vi "Input Entry.vi"(8 "error in (no error)":errorcluster, 9 "Project In":refnum<class "Project.lvclass">, 11 "Input Control":T2) -> (0 "error out":errorcluster)   [LabVIEW 2015, in "CallVIStep.lvclass"]
uses:
  CallVIStep.lvclass
  VI Input Control Typedef.ctl
  VI Input Type Typedef.ctl
  Project.lvclass
  SerializableObject/CONFIGURE_UI_STATE.ctl
  Editor/Editor.lvclass
panel:
  in  "Unsupport Type":string caption="_STRING"
  in  "Variable Name":string(combo)
  in  "Input Type":T1
  in  "_DAQmx":refnum<k21>
  in  "_COMBO_BOX":string(combo)
  in  "_ENUM":enum16{""}(ring)
  in  "_VISA":refnum<visa-resource-name>
  in  "_COLOR_BOX":u32(colorbox)
  in  "_RING":u16(ring)=5 items=["Text"=5, "ColorBox"=7, "Path"=11, "Numeric"=17, "Digital"=18, "String"=27, "IOName"=28, "ComboBox"=29, "Enum"=35, "DAQName"=49, "VISAName"=50]
  in  "_BOOLEAN":bool
  in  "_PATH":path
  in  "_NUMERIC":dbl
  in  "_STRING":string
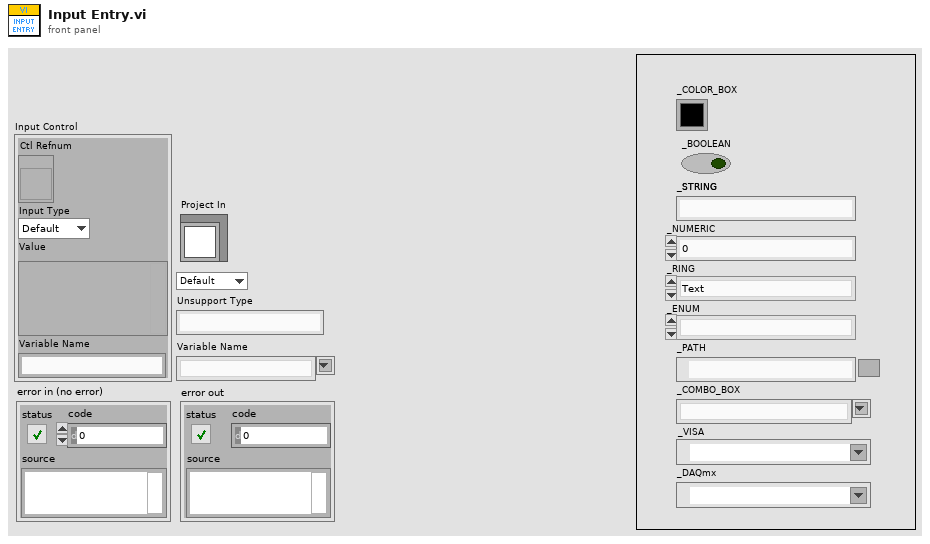
[diagram p1: front panel]
types:
  T1 = typedef "CallVIStep.lvclass/VI Input Type Typedef.ctl" = enum16{"Default", "Value", "Variable"}
  T2 = typedef "CallVIStep.lvclass/VI Input Control Typedef.ctl" = cluster{"Ctl Refnum":refnum<vi>, "Input Type":T1, "Value":variant, "Variable Name":string}
  T3 = cluster{"VI Refnum":refnum<vi>, "Input Type Refnum":refnum<vi>, "Variable Name Refnum":refnum<vi>, "Unsupport Type Refnum":refnum<vi>}
  T4 = typedef "Editor.lvclass/CONFIGURE_UI_STATE.ctl" = enum16{"UI_LOOP", "INIT", "END", "CHANGE_PANEL"}
  T5 = typedef "LVRectTypeDef.ctl" = cluster{"Left":i16, "Top":i16, "Right":i16, "Bottom":i16}
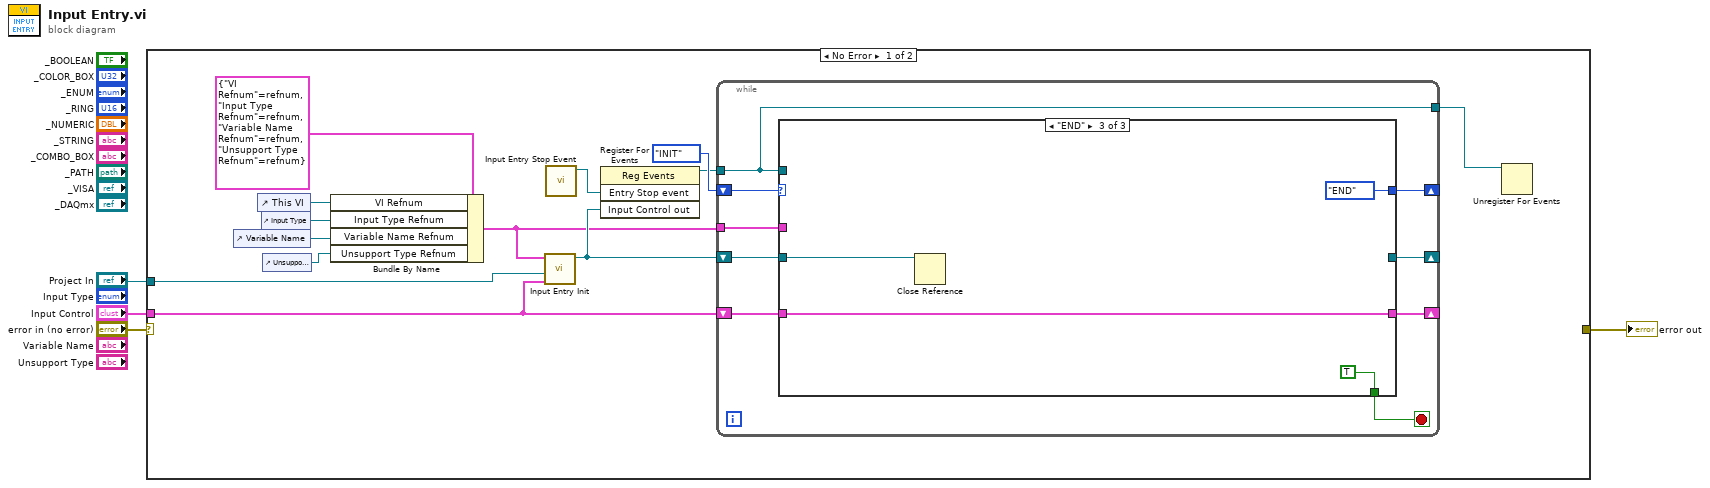
[diagram p0: block diagram]
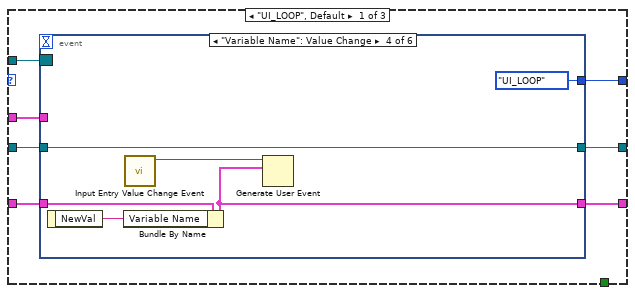
[diagram p2: hidden frame]
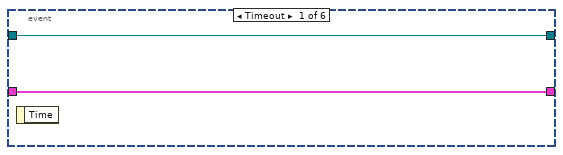
[diagram p3: hidden frame]
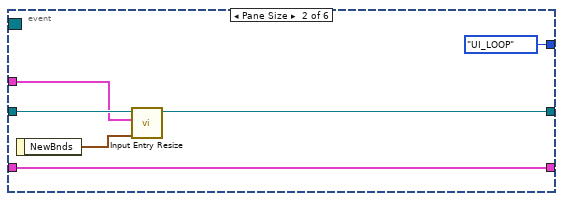
[diagram p4: hidden frame]
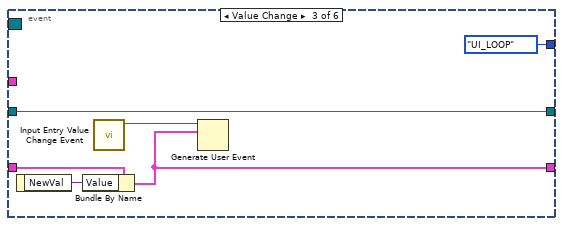
[diagram p5: hidden frame]
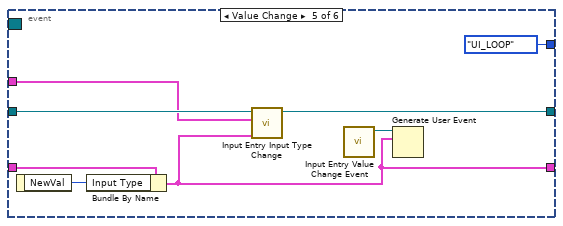
[diagram p6: hidden frame]
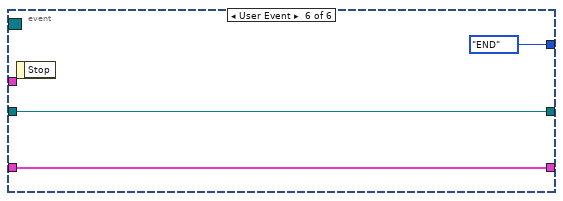
[diagram p7: hidden frame]
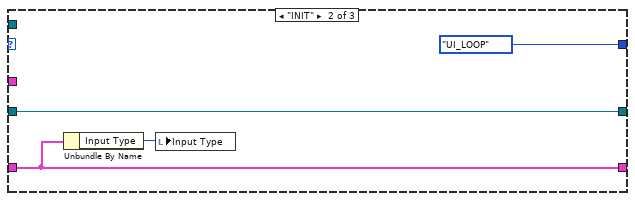
[diagram p8: hidden frame]
diagram:
  n1 = case shown="No Error" "error in (no error)" {
    selector: "error in (no error)" -> [_ w73]
    tunnel: [_ w73] -> w3
    tunnel: "Input Control" -> [w11 _]
    tunnel: "Project In" -> [w12 _]
    frame No Error {
      n2 = control-ref of="Variable Name"() -> (w7:refnum<vi>)
      n3 = control-ref of="This VI"() -> (w9:refnum<vi>)
      n4 = control-ref of="Input Type"() -> (w8:refnum<vi>)
      n5 = control-ref of="Unsupport Type"() -> (w6:refnum<vi>)
      n6 = Bundle By Name(cluster=T3 {"VI Refnum"=refnum, "Input Type Refnum"=refnum, "Variable Name Refnum"=refnum, "Unsupport Type Refnum"=refnum} ("Refnums"), "VI Refnum"=w9, "Input Type Refnum"=w8, "Variable Name Refnum"=w7, "Unsupport Type Refnum"=w6) -> (w5:T3)
      n7 = call "Input Entry Init.vi"("Input Control"=w11, "Project In"=w12, "Refnums"=w5) -> ("Input Control out"=w13:refnum<vi>)  [unwired: 8 in]
      n8 = call "Input Entry Stop Event.vi"() -> ("Entry Stop event"=w16:refnum<user-event>)  [unwired: 11 in]
      n9 = register-events(w16, w13) -> (reference out=w15:refnum<event-registration>)  [unwired: 2 in, 1 out]
      n10 = while {
        shift-right: [w25] -> _
        shift-left: CONFIGURE_UI_STATE."INIT" -> [w26]
        tunnel: w15 -> [w22]
        tunnel: [w22] -> w14
        shift-right: [w20] -> _
        shift-left: w13 -> [w21]
        shift-right: [w19] -> _
        shift-left: w11 -> [w23]
        tunnel: w5 -> [w18]
        stop <- w24 stop-if-true
        n11 = case shown="\"END\"" w26 {
          tunnel: [w33 CONFIGURE_UI_STATE."UI_LOOP" CONFIGURE_UI_STATE."END"] -> w25
          tunnel: [_ _ TRUE] -> w24
          tunnel: w23 -> [w29 w65 w69]
          tunnel: w22 -> [w32 _ _]
          tunnel: w21 -> [w31 w67 w70]
          tunnel: [w30 w67 _] -> w20
          tunnel: [w28 w65 w69] -> w19
          tunnel: w18 -> [w27 _ _]
          frame "UI_LOOP", Default {
            n12 = event shown="[3] \"Variable Name\": Value Change" {
              selector: w32 -> [_ _ _ _ _ _]
              dyn-events: _ -> [_ _ _ _ _ _]
              timeout: _ -> [_ _ _ _ _ _]
              tunnel: [_ CONFIGURE_UI_STATE."UI_LOOP" CONFIGURE_UI_STATE."UI_LOOP" CONFIGURE_UI_STATE."UI_LOOP" CONFIGURE_UI_STATE."UI_LOOP" CONFIGURE_UI_STATE."END"] -> w33
              tunnel: w31 -> [w35 w41 w47 w53 w59 w63]
              tunnel: [w35 w40 w47 w53 w58 w63] -> w30
              tunnel: w29 -> [w34 w37 w46 w52 w56 w62]
              tunnel: [w34 w37 w42 w48 w55 w62] -> w28
              tunnel: w27 -> [_ w36 _ _ w54 _]
              event Timeout {
                n13 = event-data() -> ()  [unwired: 1 in, 1 out]
              }
              event Pane Size {
                n14 = event-data() -> ("NewBnds"=w38:T5)  [unwired: 1 in]
                n15 = call "Input Entry Resize.vi"("NewBnds"=w38, "Refnums"=w36, "Control Refnum in"=w41) -> ("Control Refnum out"=w40:refnum<vi>)  [unwired: 8 in]
              }
              event Value Change {
                n16 = event-data() -> ("NewVal"=w45:variant)  [unwired: 1 in]
                n17 = Bundle By Name(cluster=w46, "Value"=w45) -> (w42:T2)
                n18 = call "Input Entry Value Change Event.vi"() -> ("Entry Value Change Event"=w44:refnum<user-event>)  [unwired: 11 in]
                n19 = Generate User Event(user event=w44, event data cluster=w42) -> ()  [unwired: 2 in, 2 out]
              }
              event "Variable Name": Value Change {
                n20 = event-data() -> ("NewVal"=w51:string)  [unwired: 1 in]
                n21 = Bundle By Name(cluster=w52, "Variable Name"=w51) -> (w48:T2)
                n22 = call "Input Entry Value Change Event.vi"() -> ("Entry Value Change Event"=w50:refnum<user-event>)  [unwired: 11 in]
                n23 = Generate User Event(user event=w50, event data cluster=w48) -> ()  [unwired: 2 in, 2 out]
              }
              event Value Change {
                n24 = event-data() -> ("NewVal"=w57:T1)  [unwired: 1 in]
                n25 = Bundle By Name(cluster=w56, "Input Type"=w57) -> (w55:T2)
                n26 = call "Input Entry Input Type Change.vi"("Input"=w55, "Refnums"=w54, "Input Control Refnum"=w59) -> ("Input Control Refnum out"=w58:refnum<vi>)  [unwired: 8 in]
                n27 = call "Input Entry Value Change Event.vi"() -> ("Entry Value Change Event"=w61:refnum<user-event>)  [unwired: 11 in]
                n28 = Generate User Event(user event=w61, event data cluster=w55) -> ()  [unwired: 2 in, 2 out]
              }
              event User Event {
                n29 = event-data() -> ()  [unwired: 1 in, 1 out]
              }
            }
          }
          frame "INIT" {
            n30 = Unbundle By Name(w65) -> ("Input Type"=w66:T1)
            n31 = local write "Input Type"(w66) -> ()
          }
          frame "END" {
            n32 = Close Reference(reference=w70) -> ()  [unwired: 1 in, 1 out]
          }
        }
      }
      n33 = Unregister For Events(event registration refnum=w14) -> ()  [unwired: 1 in, 1 out]
    }
    frame Error {
    }
  }
  "error out" <- w3
